vi "SSL Detection Ball.vi"(5 "Time Stamp":timestamp, 8 "error in":errorcluster, 9 "Array":u8[](array[numeric]) format="%02x") -> (0 "error out":errorcluster, 1 "Length-delimited":u8[](array[numeric]) format="%02x", 3 "Detection Ball":T1)   [LabVIEW 2017]
uses:
  Varint Decoder uint32.vi
  SSL Detection Ball.ctl
  <vilib>/Analysis/Matrix/Datatypes/RealMatrix.ctl
  <vilib>/Analysis/Matrix/NI_Matrix.lvlib
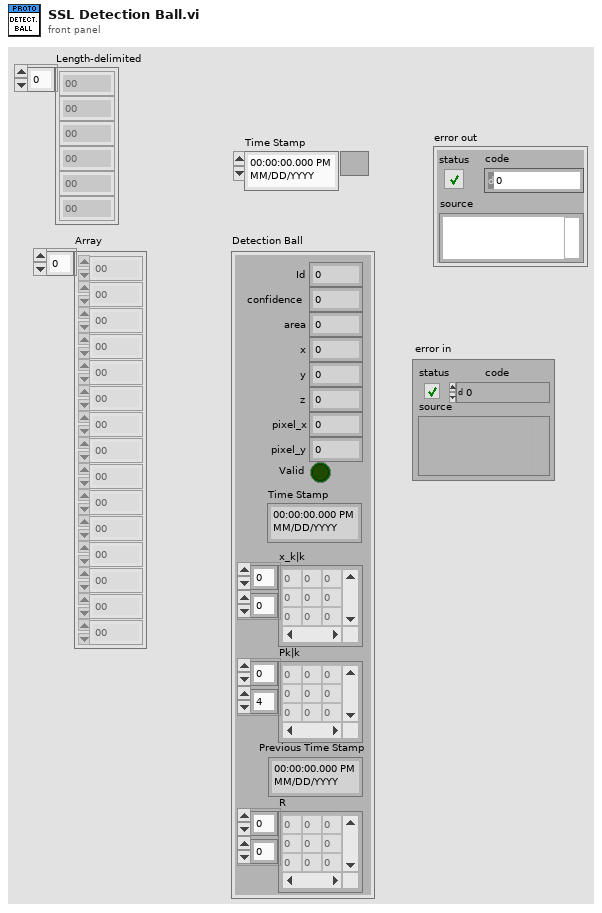
[diagram p1: front panel]
types:
  T1 = typedef "SSL Detection Ball.ctl" = cluster{"x":sgl, "area":u32, "confidence":sgl, "y":sgl, "z":sgl, "pixel_x":sgl, "pixel_y":sgl, "Valid":bool, "Time Stamp":timestamp, "x_k|k":T2, "Pk|k":T2, "Id":u32, "Previous Time Stamp":timestamp, "R":T2}
  T2 = typedef "NI_Matrix.lvlib/RealMatrix.ctl" = dbl[][]
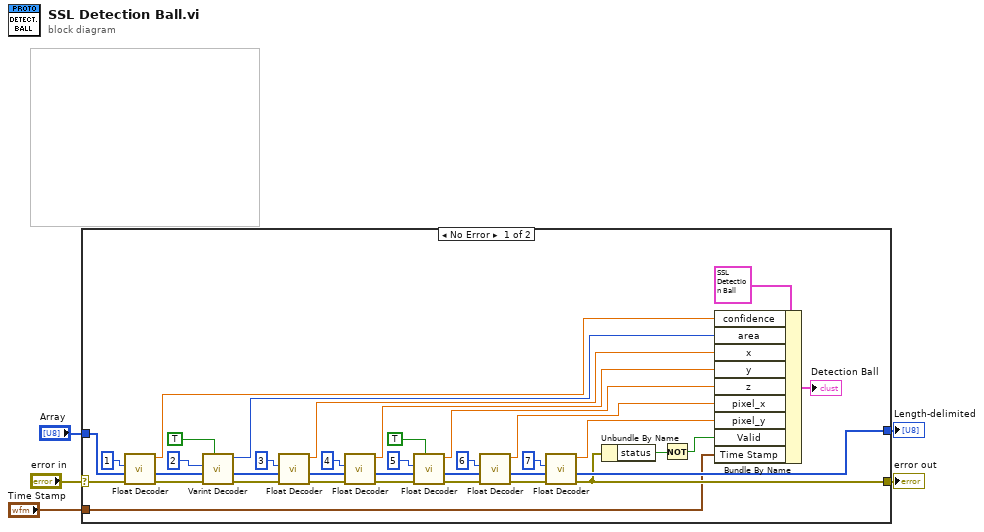
[diagram p0: block diagram]
diagram:
  n1 = case shown="No Error" "error in" {
    selector: "error in" -> [w41 w44]
    tunnel: [w10 w44] -> w4
    tunnel: [w28 w43] -> w3
    tunnel: "Array" -> [w12 w43]
    tunnel: "Time Stamp" -> [w6 _]
    frame No Error {
      n2 = call "Float Decoder.vi"("error in (no error)"=w41, "Array"=w12, "Key"=1) -> ("error out"=w40:errorcluster, "array w/ subset deleted"=w13:u8[], "Float"=w27:sgl)  [unwired: 5 in, 1 out]
      n3 = call-poly "Varint Decoder.vi"("Optional"=TRUE, "error in (no error)"=w40, "Array"=w13, "Key"=2) -> ("error out"=w39:errorcluster, "array w/ subset deleted"=w14:u8[], "Varint"=w26:u32)  [unwired: 4 in, 1 out]
      n4 = call "Float Decoder.vi"("error in (no error)"=w39, "Array"=w14, "Key"=3) -> ("error out"=w38:errorcluster, "array w/ subset deleted"=w15:u8[], "Float"=w25:sgl)  [unwired: 5 in, 1 out]
      n5 = call "Float Decoder.vi"("error in (no error)"=w38, "Array"=w15, "Key"=4) -> ("error out"=w33:errorcluster, "array w/ subset deleted"=w16:u8[], "Float"=w24:sgl)  [unwired: 5 in, 1 out]
      n6 = call "Float Decoder.vi"("Optional"=TRUE, "error in (no error)"=w33, "Array"=w16, "Key"=5) -> ("error out"=w31:errorcluster, "array w/ subset deleted"=w18:u8[], "Float"=w23:sgl)  [unwired: 4 in, 1 out]
      n7 = call "Float Decoder.vi"("error in (no error)"=w31, "Array"=w18, "Key"=6) -> ("error out"=w29:errorcluster, "array w/ subset deleted"=w19:u8[], "Float"=w7:sgl)  [unwired: 5 in, 1 out]
      n8 = call "Float Decoder.vi"("error in (no error)"=w29, "Array"=w19, "Key"=7) -> ("error out"=w10:errorcluster, "array w/ subset deleted"=w28:u8[], "Float"=w22:sgl)  [unwired: 5 in, 1 out]
      n9 = Unbundle By Name(w10) -> ("status"=w9:bool)
      n10 = Not(x=w9) -> (.not. x?=w8:bool)
      n11 = Bundle By Name(cluster=T1 {"x"=0.0, "area"=0, "confidence"=0.0, "y"=0.0, "z"=0.0, "pixel_x"=0.0, "pixel_y"=0.0, "Valid"=FALSE, "Time Stamp"=timestamp(0 s since 1904-01-01), "x_k|k"=[], "Pk|k"=[], "Id"=0, "Previous Time Stamp"=timestamp(0 s since 1904-01-01), "R"=[]} ("Detection Ball 2"), "confidence"=w27, "area"=w26, "x"=w25, "y"=w24, "z"=w23, "pixel_x"=w7, "pixel_y"=w22, "Valid"=w8, "Time Stamp"=w6) -> (→"Detection Ball":T1)
    }
    frame Error {
    }
  }
  "error out" <- w4
  "Length-delimited" <- w3
